vi "版本判断.vi"(7 "Extern":bool, 11 "固件版本号":string) -> (3 "仪器版本":T1)   [LabVIEW 2022 SP3, in "斯坦道通用流路CODmn.lvlib"]
uses:
  <vilib>/regexp/Match Regular Expression.xnode
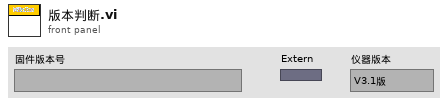
[diagram p1: front panel]
types:
  T1 = typedef "SingleStepTestV3.lvlib/SingleStepTestV3.lvclass/仪器版本.ctl" = enum16{"V3.1版", "V4版", "V3版", "V4.2版"}
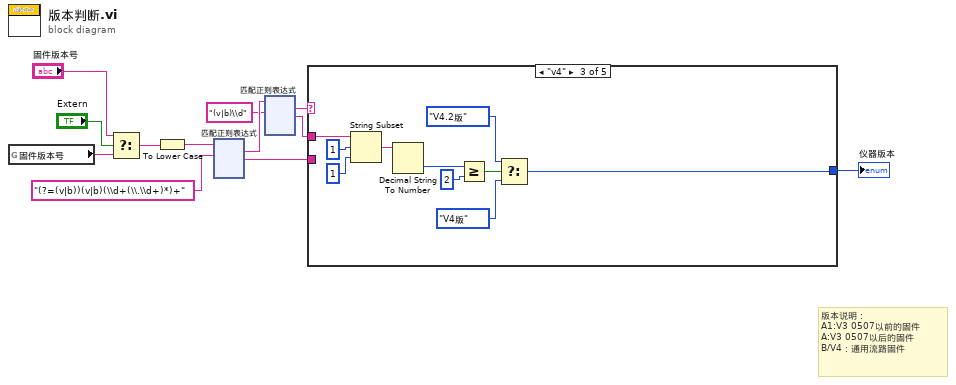
[diagram p0: block diagram]
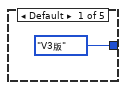
[diagram p2: hidden frame]
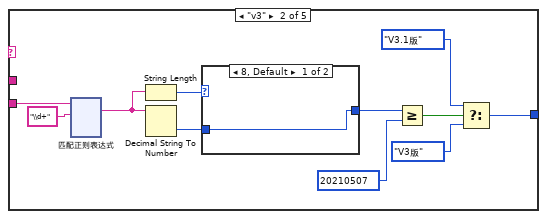
[diagram p3: hidden frame]
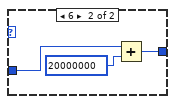
[diagram p4: hidden frame]
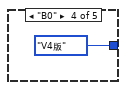
[diagram p5: hidden frame]
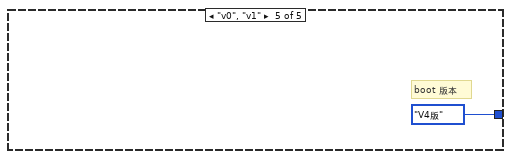
[diagram p6: hidden frame]
diagram:
  # "版本说明：\nA1:V3 0507以前的固件\nA:V3 0507以后的固件\nB/V4：通用流路固件"
  n1 = global read "VAR总磷总氮全局变量.vi" "固件版本号"() -> (w10:string)
  n2 = Select(t="固件版本号", s="Extern", f=w10) -> (s? t:f=w8:string)
  n3 = To Lower Case(string=w8) -> (all lower case string=w7:string)
  n4 = xnode "匹配正则表达式"("input string"=w7, "regular expression"="(?=(v|b))(v|b)(\\d+(\\.\\d+)*)+" ("正则表达式")) -> ("whole match"=w6:string, "after match"=w3:string)  [unwired: 4 in, 3 out]
  n5 = xnode "匹配正则表达式"("input string"=w6, "regular expression"="(v|b)\\d" ("正则表达式")) -> ("whole match"=w4:string, "after match"=w2:string)  [unwired: 4 in, 3 out]
  n6 = case shown="\"v4\"" w4 {
    tunnel: w3 -> [_ w23 _ _ _]
    tunnel: w2 -> [_ _ w154 _ _]
    tunnel: [仪器版本."V3版" ("仪器版本") w15 w147 仪器版本."V4版" ("仪器版本") 仪器版本."V4版" ("仪器版本")] -> w1
    frame Default {
    }
    frame "v3" {
      n7 = xnode "匹配正则表达式"("input string"=w23, "regular expression"="\\d+" ("正则表达式")) -> ("whole match"=w21:string)  [unwired: 4 in, 4 out]
      n8 = String Length(string=w21) -> (length=w22:i32)
      n9 = Decimal String To Number(string=w21) -> (number=w20:i32)  [unwired: 2 in, 1 out]
      n10 = case shown="8, Default" w22 {
        tunnel: w20 -> [w25 w28]
        tunnel: [w25 w26] -> w19
        frame 8, Default {
        }
        frame 6 {
          n11 = Add(x=w28, y=20000000) -> (x+y=w26:i32)
        }
      }
      n12 = Greater Or Equal?(x=w19, y=20210507) -> (x >= y?=w17:bool)
      n13 = Select(t=仪器版本."V3.1版" ("仪器版本"), s=w17, f=仪器版本."V3版") -> (s? t:f=w15:T1)
    }
    frame "v4" {
      n14 = String Subset(string=w154, offset (0)=1 ("偏移量(0)"), length (rest)=1 ("长度（剩余）")) -> (substring=w153:string)
      n15 = Decimal String To Number(string=w153) -> (number=w152:i32)  [unwired: 2 in, 1 out]
      n16 = Greater Or Equal?(x=w152, y=2) -> (x >= y?=w150:bool)
      n17 = Select(t=仪器版本."V4.2版" ("仪器版本"), s=w150, f=仪器版本."V4版" ("仪器版本")) -> (s? t:f=w147:T1)
    }
    frame "B0" {
    }
    frame "v0", "v1" {
      # "boot 版本"
    }
  }
  "仪器版本" <- w1
